vi "Tester serv.vi"() -> ()   [LabVIEW 2026]
uses:
  <vilib>/MakerHub/LINX/Public/Utilities/Open Serial.vi
  <vilib>/MakerHub/LINX/LMH-LINX.lvlib
panel:
  in  "Knob":u8(knob) scale=100.0..600.0
  in  "PALEC":u8
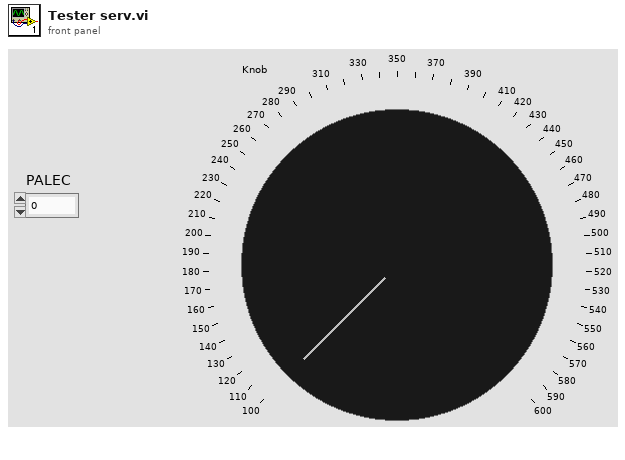
[diagram p1: front panel]
types:
  T1 = typedef "LMH-LINX.lvlib/LINX Ref.ctl" = cluster{"IO":T2, "Interface":T3, "LINX Device Config":T4}
  T2 = typedef "LMH-LINX.lvlib/Platform.ctl" = enum16{"Remote", "Local"}
  T3 = typedef "LMH-LINX.lvlib/Interface.ctl" = enum16{"Serial", "TCP"}
  T4 = typedef "LMH-LINX.lvlib/Device.lvlib/LINX Device Config.ctl" = cluster{"Interface":T3, "COM Port":refnum<visa-resource-name>, "TCP Configuration":T5, "Device Family":u8, "Device ID":u8, "Device Name":string, "TCP Ref":refnum<k5>, "Channels":T6}
  T5 = typedef "LMH-LINX.lvlib/Device.lvlib/TCP Config.ctl" = cluster{"IP Address":string, "Port":u16}
  T6 = typedef "LMH-LINX.lvlib/Channels.ctl" = cluster{"DI":u8[], "DO":u8[], "AI":u8[], "AO":u8[], "PWM":u8[], "QE":u8[], "UART":u8[], "I2C 2":u8[], "SPI":u8[], "CAN":u8[], "Servo":u8[], "AI Ref (V)":dbl, "AI Resolution (Bits)":u8, "AO Ref (V)":dbl, "AO Resolution (Bits)":u8}
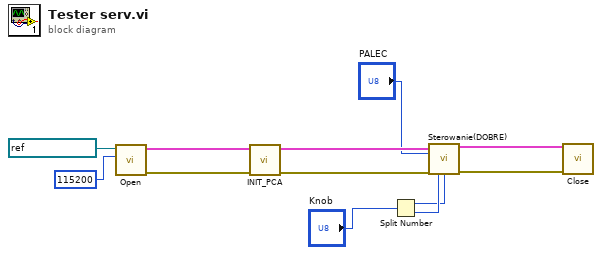
[diagram p0: block diagram]
diagram:
  n1 = call-poly <vilib>:"Open.vi"("Baud Rate Override"=u32 115200, "Serial Port"=refnum<visa-resource-name> "COM3") -> ("Error Out"=w9:errorcluster, "LINX Resource"=w10:T1)  [unwired: 7 in, 1 out]
  n2 = call "INIT_PCA.vi"("Error In"=w9, "LINX Resource 2"=w10) -> ("error out"=w7:errorcluster, "LINX Resource"=w8:T1)  [unwired: 8 in]
  n3 = Split Number(x="Knob") -> (hi(x)=w3:u8, lo(x)=w4:u8)
  n4 = call "Sterowanie(DOBRE).vi"("LINX Resource in"=w8, "element"="PALEC", "error in (no error)"=w7, "element 4"=w4, "element 5"=w3) -> ("LINX Resource out"=w2:T1, "error out"=w1:errorcluster)  [unwired: 9 in]
  n5 = call <vilib>:"Close.vi"("Error In"=w1, "LINX Resource"=w2) -> ()  [unwired: 9 in, 1 out]
